vi "LWXPS_ControllerMotionKernelMinMaxTimeLoadGet.vi"(1 "XPS Reference IN":refnum<k24>, 4 "LabVIEW error IN":errorcluster) -> (8 "XPS Reference OUT":refnum<k24>, 9 "LabVIEW error OUT":errorcluster, 10 "Returned error code":i32, 11 "XPS Error String":string, 12 "Minimum CPU Total Load Ratio":dbl, 13 "Maximum CPU Servitudes Load Ratio":dbl, 14 "Maximum CPU Total Load Ratio":dbl, 15 "Minimum CPU Corrector Load Ratio":dbl, 16 "Maximum CPU Corrector Load Ratio":dbl, 17 "Minimum CPU Profiler Load Ratio":dbl, 18 "Maximum CPU Profiler Load Ratio":dbl, 19 "Minimum CPU Servitudes Load Ratio":dbl)   [LabVIEW 2014]
uses:
  D:/XPSQ8_LabView_Library/Development/Source/Dll/Newport.XPS.CommandInterface.dll
  Dll/Newport.XPS.CommandInterface.dll
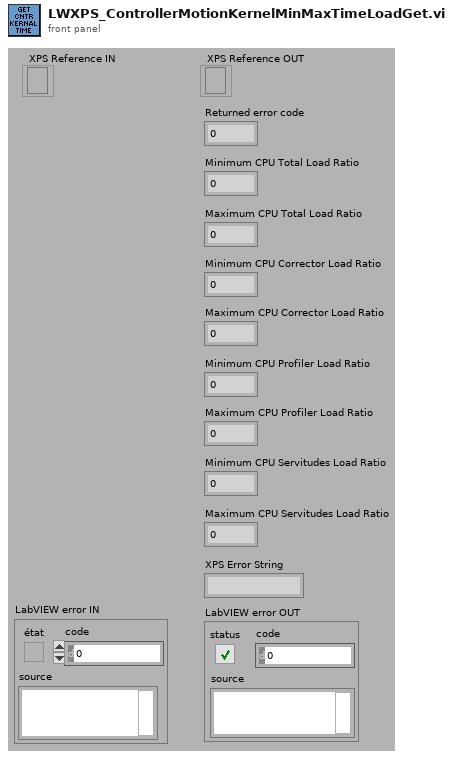
[diagram p1: front panel]
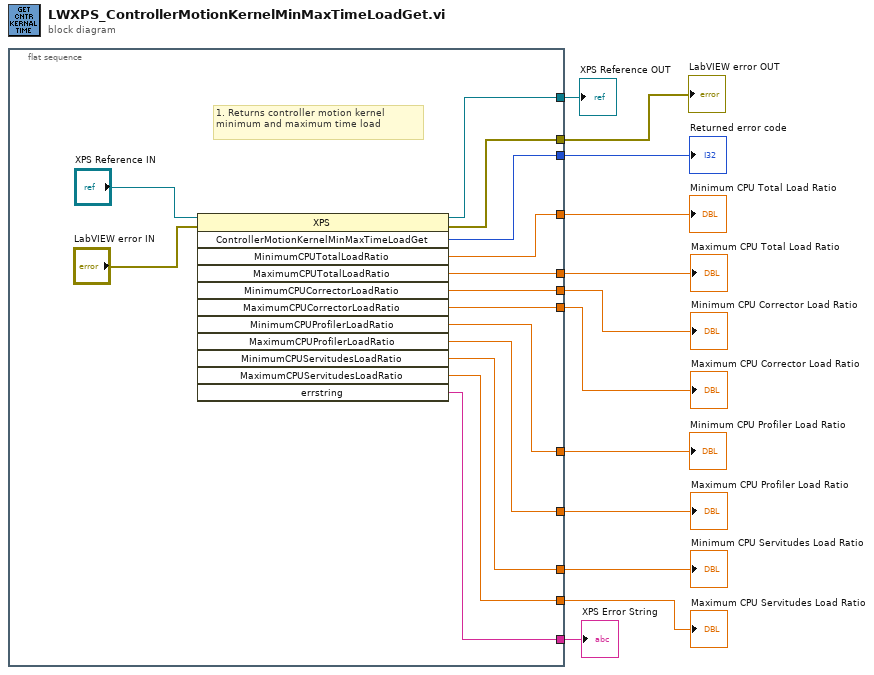
[diagram p0: block diagram]
diagram:
  n1 = flat-sequence {
    tunnel: [w23] -> w11
    tunnel: [w24] -> w12
    tunnel: [w22] -> w2
    tunnel: [w21] -> w10
    tunnel: [w19] -> w9
    tunnel: [w13] -> w8
    tunnel: [w18] -> w7
    tunnel: [w14] -> w6
    tunnel: [w20] -> w5
    tunnel: [w17] -> w4
    tunnel: [w16] -> w3
    tunnel: [w15] -> w1
    frame #0 {
      # "1. Returns controller motion kernel minimum and maximum time load"
      n2 = invoke class="XPS" method="ControllerMotionKernelMinMaxTimeLoadGet"(reference="XPS Reference IN", error in="LabVIEW error IN") -> (reference out=w23:refnum<k24>, error out=w24:errorcluster, "ControllerMotionKernelMinMaxTimeLoadGet"=w22:i32, "MinimumCPUTotalLoadRatio"=w15:dbl, "MaximumCPUTotalLoadRatio"=w21:dbl, "MinimumCPUCorrectorLoadRatio"=w20:dbl, "MaximumCPUCorrectorLoadRatio"=w19:dbl, "MinimumCPUProfilerLoadRatio"=w18:dbl, "MaximumCPUProfilerLoadRatio"=w14:dbl, "MinimumCPUServitudesLoadRatio"=w13:dbl, "MaximumCPUServitudesLoadRatio"=w17:dbl, "errstring"=w16:string)  [unwired: 10 in]
    }
  }
  "XPS Reference OUT" <- w11
  "LabVIEW error OUT" <- w12
  "Minimum CPU Total Load Ratio" <- w1
  "Maximum CPU Total Load Ratio" <- w10
  "Minimum CPU Corrector Load Ratio" <- w5
  "Maximum CPU Corrector Load Ratio" <- w9
  "Minimum CPU Servitudes Load Ratio" <- w8
  "Minimum CPU Profiler Load Ratio" <- w7
  "Maximum CPU Profiler Load Ratio" <- w6
  "Maximum CPU Servitudes Load Ratio" <- w4
  "XPS Error String" <- w3
  "Returned error code" <- w2
